vi "Generate File Name.vi"(11 "properties":cluster{"Key":string, "Value":string}[](array[cluster])) -> (3 "Array":cluster{"Key":string, "Value":string}[](array[cluster]))   [LabVIEW 2016]
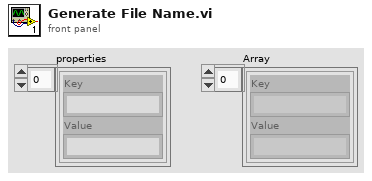
[diagram p1: front panel]
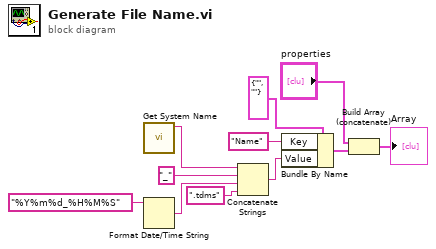
[diagram p0: block diagram]
diagram:
  n1 = call "Get System Name.vi"() -> ("name"=w1:string)  [unwired: 11 in]
  n2 = Format Date/Time String(time format string (%c)="%Y%m%d_%H%M%S") -> (date/time string=w7:string)  [unwired: 2 in]
  n3 = Concatenate Strings(w1, "_" ("string"), w7, ".tdms" ("string")) -> (w11:string)
  n4 = Bundle By Name(cluster=cluster{"Key":string, "Value":string} {"Key"="", "Value"=""} ("Property"), "Key"="Name" ("element"), "Value"=w11) -> (w3:cluster{"Key":string, "Value":string})
  n5 = Build Array (concatenate)("properties", w3) -> (→"Array":cluster{"Key":string, "Value":string}[])
